vi "UpdateUserInterface.vi"(8 "error in (no error)":errorcluster, 10 "DataExchange":T1, 11 "CameraController in":refnum<class "CameraController.lvclass">) -> (0 "error out":errorcluster, 2 "DataExchange Out":T1, 3 "CameraController out":refnum<class "CameraController.lvclass">)   [LabVIEW 2020, in "CameraController.lvlib" / "CameraController.lvclass"]
uses:
  CameraController.lvclass
  Model/Hardware Abstraction Layer/Component/Device/Device/DataExchange.ctl
  <vilib>/vision/Image Controls.llb/IMAQ Image.ctl
  CameraController.lvclass/CameraController.ctl
  Model/Hardware Abstraction Layer/Component/GenericActor/GenericActor/GenericController.lvclass
  Interface/DataListener/DataListener.lvclass
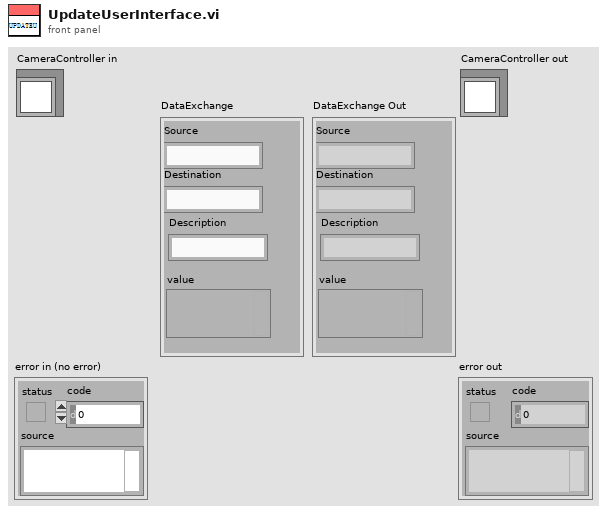
[diagram p1: front panel]
types:
  T1 = typedef "DataListener.lvclass/DataExchange.ctl" = cluster{"Source":string, "Destination":string, "Description":string, "value":variant}
  T2 = typedef "IMAQ Image.ctl" = refnum<image>
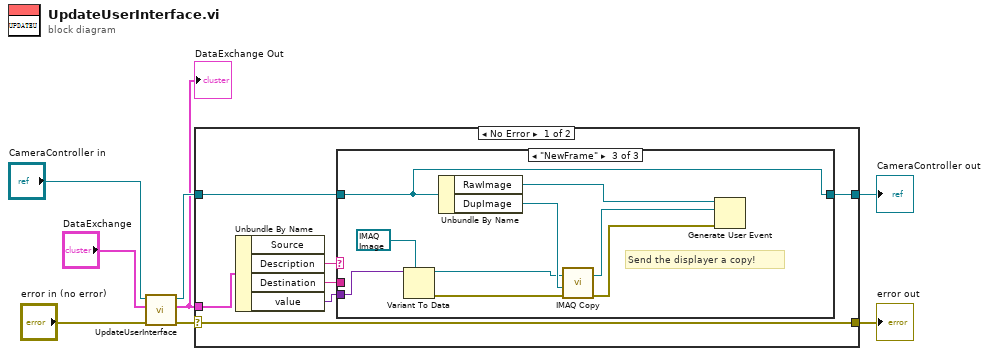
[diagram p0: block diagram]
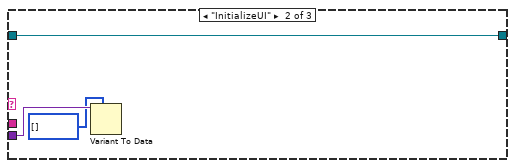
[diagram p3: hidden frame]
diagram:
  n1 = call-parent "UpdateUserInterface.vi"("error in (no error)"="error in (no error)", "DataExchange"="DataExchange", "GenericController in"="CameraController in") -> ("error out"=w4:errorcluster, "DataExchange Out"=w1:T1, "GenericController out"=w5:refnum<class "CameraController.lvclass">)  [unwired: 6 in]
  "DataExchange Out" <- w1
  n2 = case shown="No Error" w4 {
    selector: w4 -> [w15 w30]
    tunnel: [w15 w30] -> w2
    tunnel: [w9 w29] -> w3
    tunnel: w5 -> [w10 w29]
    tunnel: w1 -> [w14 _]
    frame No Error {
      n3 = Unbundle By Name(w14) -> ("Description"=w11:string, "Destination"=w12:string, "value"=w13:variant)  [unwired: 1 out]
      n4 = case shown="\"NewFrame\"" w11 {
        tunnel: w13 -> [_ w18 w28]
        tunnel: w12 -> [_ _ _]
        tunnel: w10 -> [w16 w19 w25]
        tunnel: [w16 w19 w25] -> w9
        frame Default {
        }
        frame "InitializeUI" {
          n5 = Variant To Data(type=i32[] [] ("appended array"), Variant=w18) -> ()  [unwired: 1 in, 2 out]
        }
        frame "NewFrame" {
          # "Send the displayer a copy!"
          n6 = Variant To Data(type=T2 refnum ("event data"), Variant=w28) -> (data=w21:T2, error out=w23:errorcluster)  [unwired: 1 in]
          n7 = Unbundle By Name(w25) -> ("RawImage"=w27:refnum<user-event>, "DupImage"=w24:T2)
          n8 = call "IMAQ Copy"("error in (no error)"=w23, "Image Dst"=w24, "Image Src"=w21) -> ("error out"=w22:errorcluster, "Image Dst Out"=w20:T2)  [unwired: 3 in]
          n9 = Generate User Event(user event=w27, event data cluster=w20, error in=w22) -> ()  [unwired: 1 in, 2 out]
        }
      }
    }
    frame Error {
    }
  }
  "error out" <- w2
  "CameraController out" <- w3
